vi "Clipper.vi"(8 "error in (no error)":errorcluster) -> (0 "error out":errorcluster)   [LabVIEW 2020]
doc: "This template is for the Queued Message Handler design pattern.\n\nThe Event Handling Loop generates messages based on user interface actions.\n\nThe Message Handling Loop processes messages generated by the Event Handling Loop, or by other messages. The messages are string values, so new messages can be added easily to the Message Cases case structure in the Message Handling Loop. Each message cluster can also provide an optional value for Message Data, which is a variant that can be converted to whatever message-specific data is required."
uses:
  <vilib>/Utility/miscctls.llb/LVCursorListTypeDef.ctl
  Analysis Support/Controls/UI Data-Clipper.ctl
  Collection Support/Message Queue/Enqueue Message (Single).vi
  Collection Support/Message Queue/Enqueue Message (Array).vi
  <vilib>/Utility/error.llb/Error Cluster From Error Code.vi
  <vilib>/ErrorRing/Error Ring.xnode
panel:
  in  "Stop Everything?":bool
  out "Right":dbl
  out "Left":dbl
  out "Flow":dynamicdata(graph)
  out "Pressure":dynamicdata(graph)
  out "Audio":dynamicdata(graph)
  out "File Name Display":string
  in  "Remove":bool
  in  "Set Cursors":bool
  in  "Edit File":bool
  out "Message":string
  in  "Save":bool
  in  "Open":bool
  in  "Exit":bool
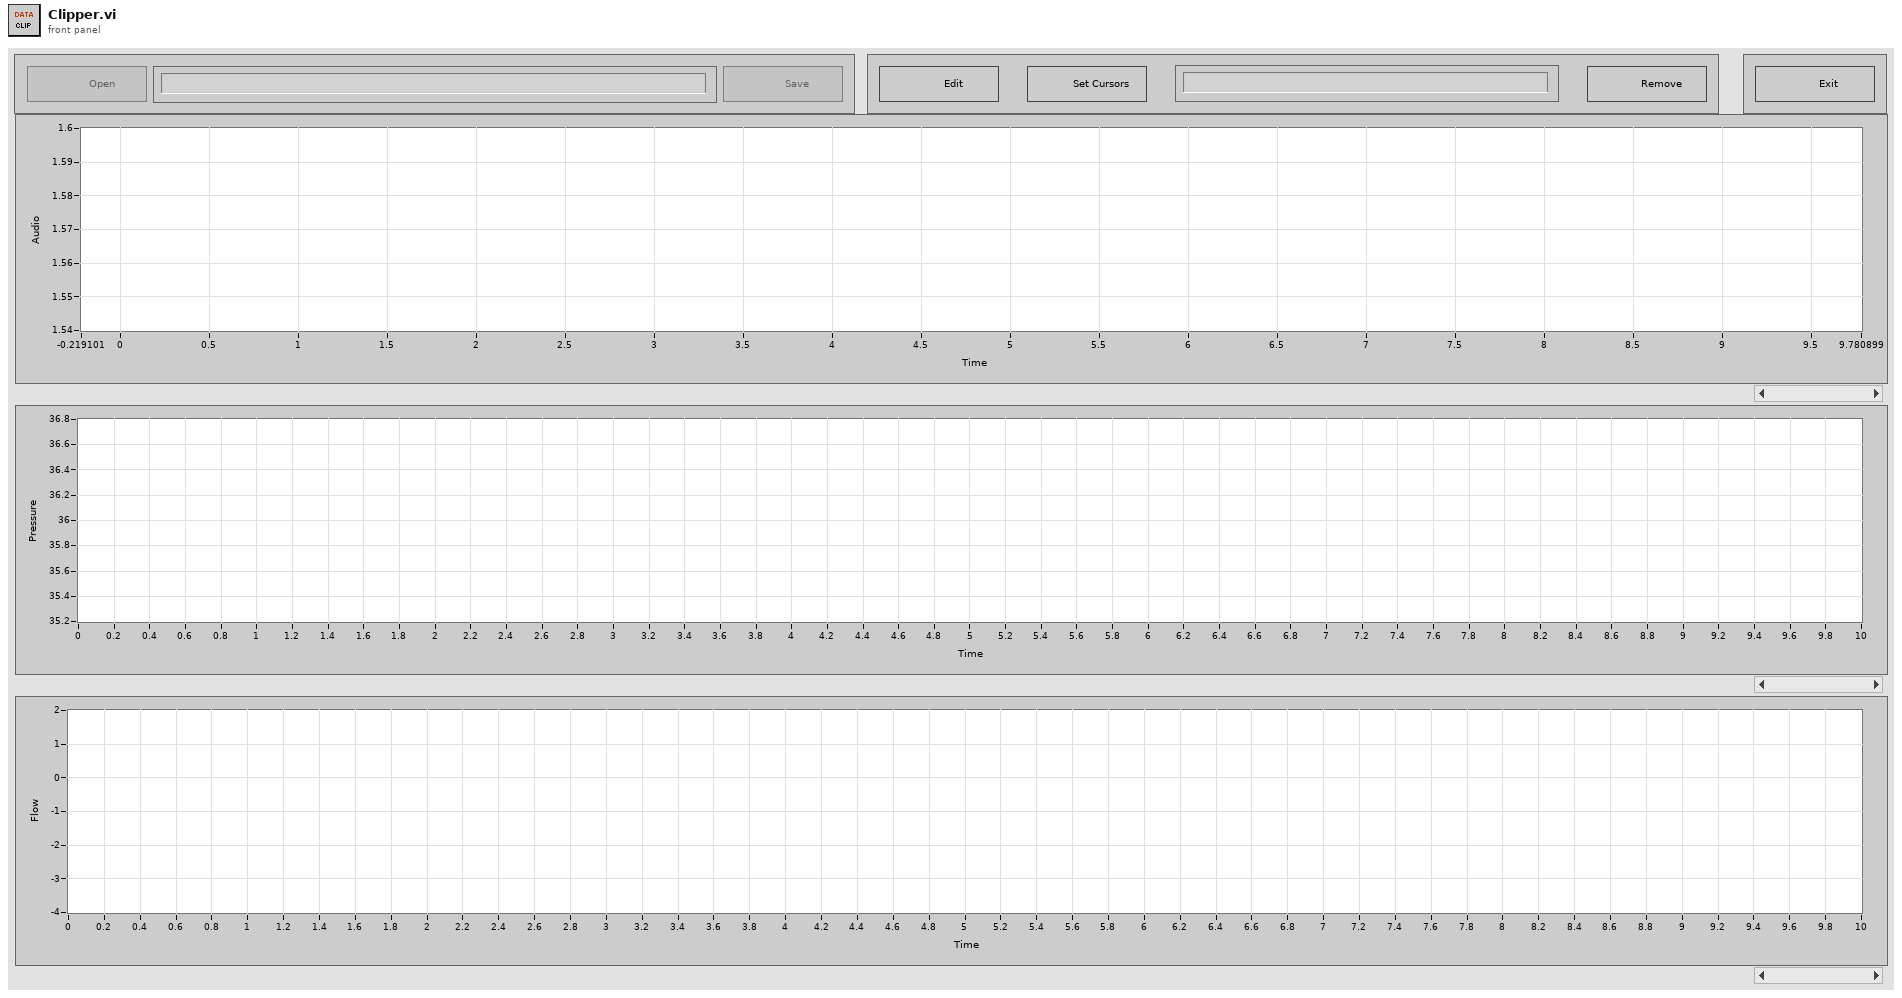
[diagram p1: front panel]
types:
  T1 = typedef "UI Data-Clipper.ctl" = cluster{"File Loaded?":bool, "Message":string, "Open Ref":refnum<vi>, "Save Ref":refnum<vi>, "Message Ref":refnum<vi>, "Exit Button Ref":refnum<vi>, "Remove Ref":refnum<vi>, "Set Cursors Ref":refnum<vi>, "Edit File Ref":refnum<vi>, "Audio Ref":refnum<vi>, "Pressure Ref":refnum<vi>, "Flow Ref":refnum<vi>, "Audio":dynamicdata, "Pressure":dynamicdata, "Flow":dynamicdata, "Left Cursor Position":dbl, "Right Cursor Position":dbl, "Cursors Locked?":bool, "File Name Display":string}
  T2 = typedef "LVCursorListTypeDef.ctl" = cluster{"Name":string, "Color":u32, "Style":u8, "Point Style":u8, "Name Visible":bool, "Allow Drag":bool, "Cursor Mode":u32, "Plot":i32, "Index":i32, "Position":cluster{"X":dbl, "Y":dbl}, "X Scale":u32, "Y Scale":u32, "Watch Plots":i32[], "Watch All Plots":bool, "Plot Area":i32, "Label Offset":cluster{"X":dbl, "Y":dbl}}[]
  T3 = typedef "All Message Queues.ctl" = cluster{"UI":refnum<queue>}
  T4 = cluster{"Cursor Constants[0]":cluster{"Name":string, "Color":u32, "Style":u8, "Point Style":u8, "Name Visible":bool, "Allow Drag":bool, "Cursor Mode":u32, "Plot":i32, "Index":i32, "Position":cluster{"X":dbl, "Y":dbl}, "X Scale":u32, "Y Scale":u32, "Watch Plots":i32[], "Watch All Plots":bool, "Plot Area":i32, "Label Offset":cluster{"X":dbl, "Y":dbl}}, "Cursor Constants[1]":cluster{"Name":string, "Color":u32, "Style":u8, "Point Style":u8, "Name Visible":bool, "Allow Drag":bool, "Cursor Mode":u32, "Plot":i32, "Index":i32, "Position":cluster{"X":dbl, "Y":dbl}, "X Scale":u32, "Y Scale":u32, "Watch Plots":i32[], "Watch All Plots":bool, "Plot Area":i32, "Label Offset":cluster{"X":dbl, "Y":dbl}}, "Cursor Constants[2]":cluster{"Name":string, "Color":u32, "Style":u8, "Point Style":u8, "Name Visible":bool, "Allow Drag":bool, "Cursor Mode":u32, "Plot":i32, "Index":i32, "Position":cluster{"X":dbl, "Y":dbl}, "X Scale":u32, "Y Scale":u32, "Watch Plots":i32[], "Watch All Plots":bool, "Plot Area":i32, "Label Offset":cluster{"X":dbl, "Y":dbl}}, "Cursor Constants[3]":cluster{"Name":string, "Color":u32, "Style":u8, "Point Style":u8, "Name Visible":bool, "Allow Drag":bool, "Cursor Mode":u32, "Plot":i32, "Index":i32, "Position":cluster{"X":dbl, "Y":dbl}, "X Scale":u32, "Y Scale":u32, "Watch Plots":i32[], "Watch All Plots":bool, "Plot Area":i32, "Label Offset":cluster{"X":dbl, "Y":dbl}}, "Cursor Constants[4]":cluster{"Name":string, "Color":u32, "Style":u8, "Point Style":u8, "Name Visible":bool, "Allow Drag":bool, "Cursor Mode":u32, "Plot":i32, "Index":i32, "Position":cluster{"X":dbl, "Y":dbl}, "X Scale":u32, "Y Scale":u32, "Watch Plots":i32[], "Watch All Plots":bool, "Plot Area":i32, "Label Offset":cluster{"X":dbl, "Y":dbl}}, "Cursor Constants[5]":cluster{"Name":string, "Color":u32, "Style":u8, "Point Style":u8, "Name Visible":bool, "Allow Drag":bool, "Cursor Mode":u32, "Plot":i32, "Index":i32, "Position":cluster{"X":dbl, "Y":dbl}, "X Scale":u32, "Y Scale":u32, "Watch Plots":i32[], "Watch All Plots":bool, "Plot Area":i32, "Label Offset":cluster{"X":dbl, "Y":dbl}}, "Cursor Constants[6]":cluster{"Name":string, "Color":u32, "Style":u8, "Point Style":u8, "Name Visible":bool, "Allow Drag":bool, "Cursor Mode":u32, "Plot":i32, "Index":i32, "Position":cluster{"X":dbl, "Y":dbl}, "X Scale":u32, "Y Scale":u32, "Watch Plots":i32[], "Watch All Plots":bool, "Plot Area":i32, "Label Offset":cluster{"X":dbl, "Y":dbl}}, "Cursor Constants[7]":cluster{"Name":string, "Color":u32, "Style":u8, "Point Style":u8, "Name Visible":bool, "Allow Drag":bool, "Cursor Mode":u32, "Plot":i32, "Index":i32, "Position":cluster{"X":dbl, "Y":dbl}, "X Scale":u32, "Y Scale":u32, "Watch Plots":i32[], "Watch All Plots":bool, "Plot Area":i32, "Label Offset":cluster{"X":dbl, "Y":dbl}}, "Cursor Constants[8]":cluster{"Name":string, "Color":u32, "Style":u8, "Point Style":u8, "Name Visible":bool, "Allow Drag":bool, "Cursor Mode":u32, "Plot":i32, "Index":i32, "Position":cluster{"X":dbl, "Y":dbl}, "X Scale":u32, "Y Scale":u32, "Watch Plots":i32[], "Watch All Plots":bool, "Plot Area":i32, "Label Offset":cluster{"X":dbl, "Y":dbl}}}
  T5 = cluster{"Name":string, "Color":u32, "Style":u8, "Point Style":u8, "Name Visible":bool, "Allow Drag":bool, "Cursor Mode":u32, "Plot":i32, "Index":i32, "Position":cluster{"X":dbl, "Y":dbl}, "X Scale":u32, "Y Scale":u32, "Watch Plots":i32[], "Watch All Plots":bool, "Plot Area":i32, "Label Offset":cluster{"X":dbl, "Y":dbl}}[]
  T6 = cluster{"CrsrList[0]":cluster{"Name":string, "Color":u32, "Style":u8, "Point Style":u8, "Name Visible":bool, "Allow Drag":bool, "Cursor Mode":u32, "Plot":i32, "Index":i32, "Position":cluster{"X":dbl, "Y":dbl}, "X Scale":u32, "Y Scale":u32, "Watch Plots":i32[], "Watch All Plots":bool, "Plot Area":i32, "Label Offset":cluster{"X":dbl, "Y":dbl}}, "CrsrList[1]":cluster{"Name":string, "Color":u32, "Style":u8, "Point Style":u8, "Name Visible":bool, "Allow Drag":bool, "Cursor Mode":u32, "Plot":i32, "Index":i32, "Position":cluster{"X":dbl, "Y":dbl}, "X Scale":u32, "Y Scale":u32, "Watch Plots":i32[], "Watch All Plots":bool, "Plot Area":i32, "Label Offset":cluster{"X":dbl, "Y":dbl}}, "CrsrList[2]":cluster{"Name":string, "Color":u32, "Style":u8, "Point Style":u8, "Name Visible":bool, "Allow Drag":bool, "Cursor Mode":u32, "Plot":i32, "Index":i32, "Position":cluster{"X":dbl, "Y":dbl}, "X Scale":u32, "Y Scale":u32, "Watch Plots":i32[], "Watch All Plots":bool, "Plot Area":i32, "Label Offset":cluster{"X":dbl, "Y":dbl}}, "CrsrList[3]":cluster{"Name":string, "Color":u32, "Style":u8, "Point Style":u8, "Name Visible":bool, "Allow Drag":bool, "Cursor Mode":u32, "Plot":i32, "Index":i32, "Position":cluster{"X":dbl, "Y":dbl}, "X Scale":u32, "Y Scale":u32, "Watch Plots":i32[], "Watch All Plots":bool, "Plot Area":i32, "Label Offset":cluster{"X":dbl, "Y":dbl}}, "CrsrList[4]":cluster{"Name":string, "Color":u32, "Style":u8, "Point Style":u8, "Name Visible":bool, "Allow Drag":bool, "Cursor Mode":u32, "Plot":i32, "Index":i32, "Position":cluster{"X":dbl, "Y":dbl}, "X Scale":u32, "Y Scale":u32, "Watch Plots":i32[], "Watch All Plots":bool, "Plot Area":i32, "Label Offset":cluster{"X":dbl, "Y":dbl}}, "CrsrList[5]":cluster{"Name":string, "Color":u32, "Style":u8, "Point Style":u8, "Name Visible":bool, "Allow Drag":bool, "Cursor Mode":u32, "Plot":i32, "Index":i32, "Position":cluster{"X":dbl, "Y":dbl}, "X Scale":u32, "Y Scale":u32, "Watch Plots":i32[], "Watch All Plots":bool, "Plot Area":i32, "Label Offset":cluster{"X":dbl, "Y":dbl}}, "CrsrList[6]":cluster{"Name":string, "Color":u32, "Style":u8, "Point Style":u8, "Name Visible":bool, "Allow Drag":bool, "Cursor Mode":u32, "Plot":i32, "Index":i32, "Position":cluster{"X":dbl, "Y":dbl}, "X Scale":u32, "Y Scale":u32, "Watch Plots":i32[], "Watch All Plots":bool, "Plot Area":i32, "Label Offset":cluster{"X":dbl, "Y":dbl}}, "CrsrList[7]":cluster{"Name":string, "Color":u32, "Style":u8, "Point Style":u8, "Name Visible":bool, "Allow Drag":bool, "Cursor Mode":u32, "Plot":i32, "Index":i32, "Position":cluster{"X":dbl, "Y":dbl}, "X Scale":u32, "Y Scale":u32, "Watch Plots":i32[], "Watch All Plots":bool, "Plot Area":i32, "Label Offset":cluster{"X":dbl, "Y":dbl}}, "CrsrList[8]":cluster{"Name":string, "Color":u32, "Style":u8, "Point Style":u8, "Name Visible":bool, "Allow Drag":bool, "Cursor Mode":u32, "Plot":i32, "Index":i32, "Position":cluster{"X":dbl, "Y":dbl}, "X Scale":u32, "Y Scale":u32, "Watch Plots":i32[], "Watch All Plots":bool, "Plot Area":i32, "Label Offset":cluster{"X":dbl, "Y":dbl}}}
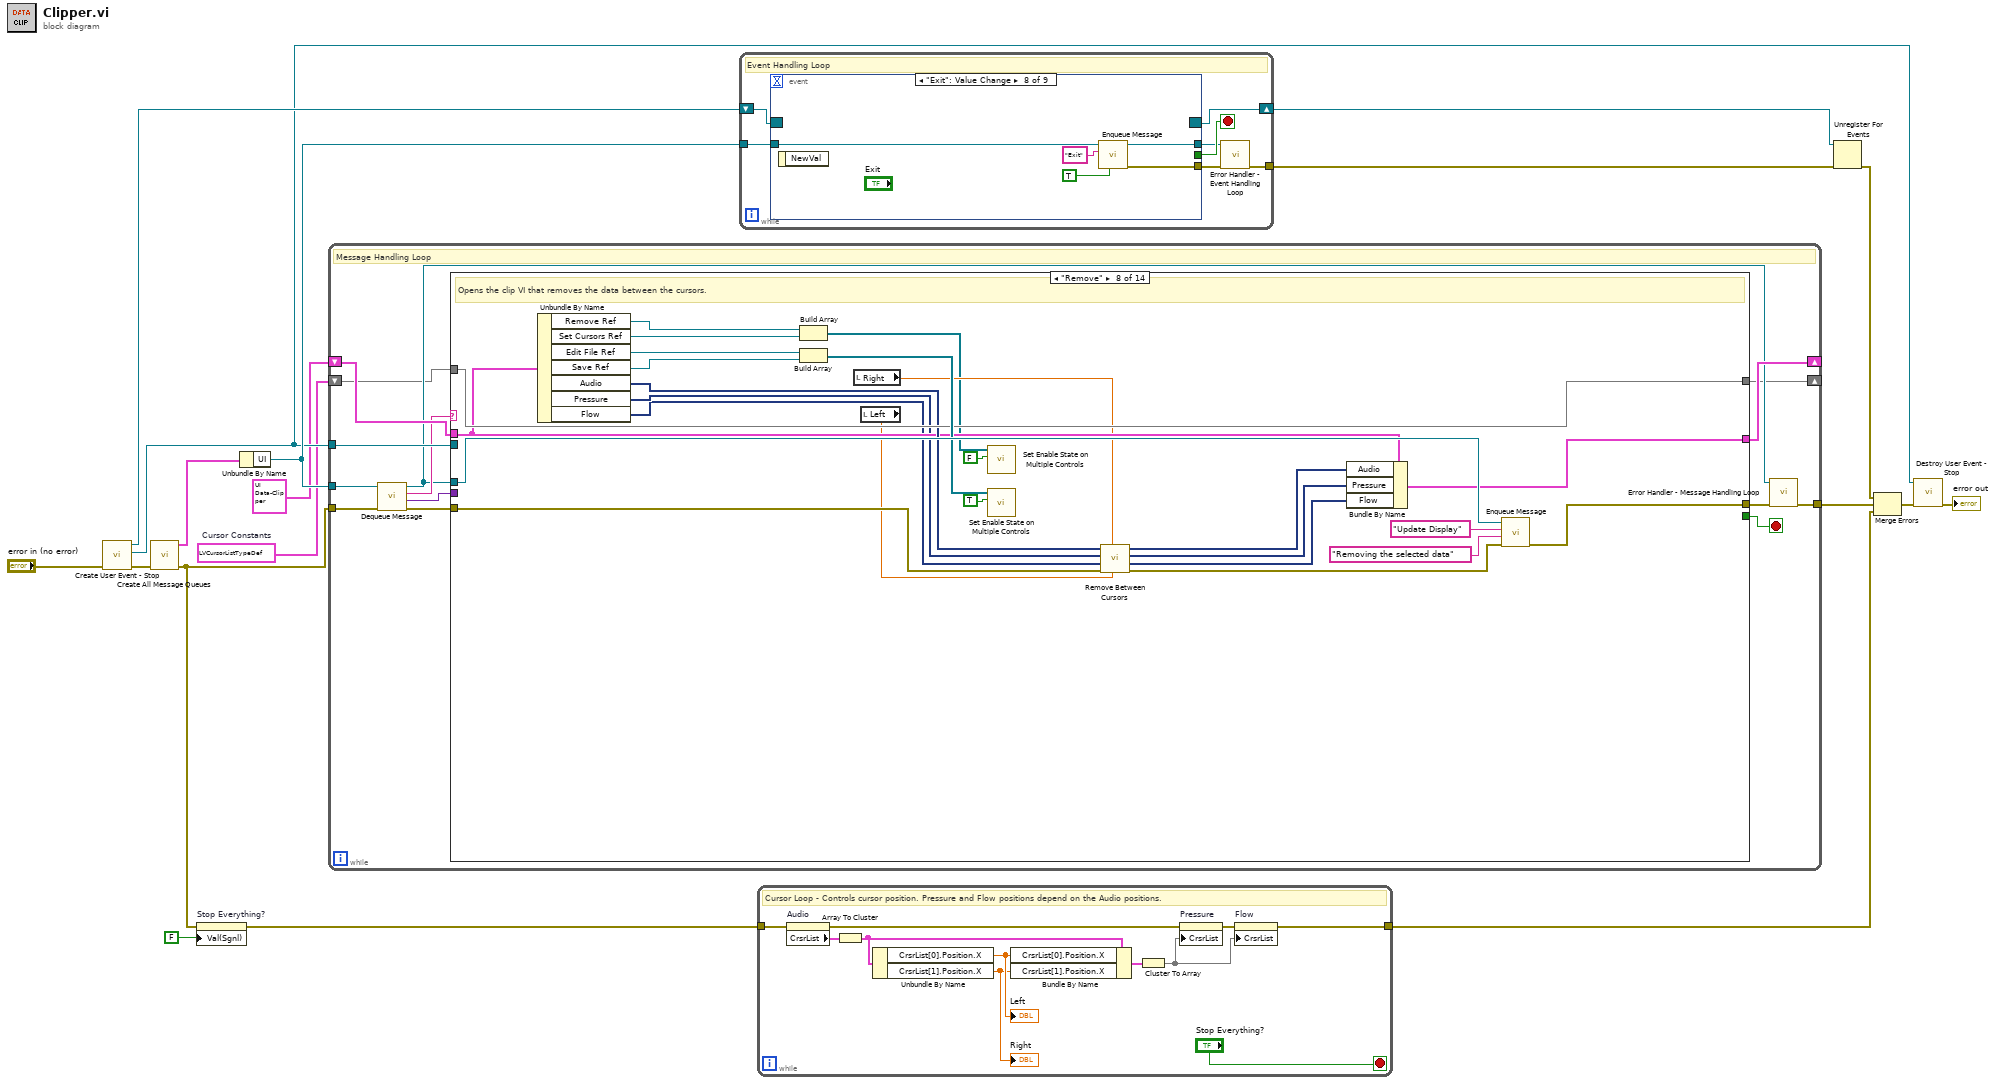
[diagram p0: block diagram]
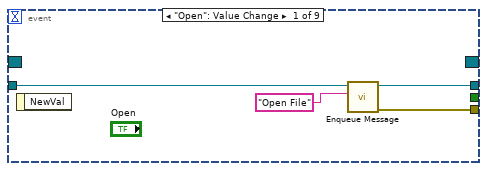
[diagram p2: hidden frame]
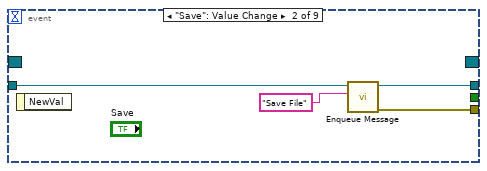
[diagram p3: hidden frame]
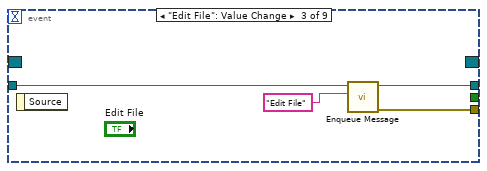
[diagram p4: hidden frame]
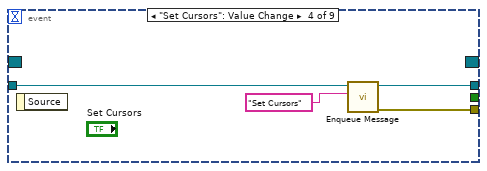
[diagram p5: hidden frame]
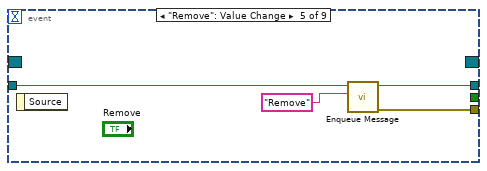
[diagram p6: hidden frame]
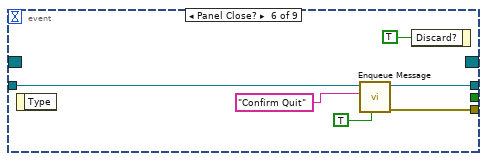
[diagram p7: hidden frame]
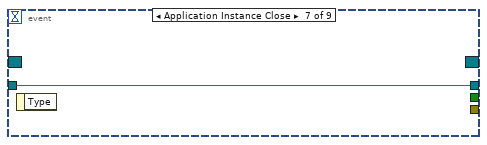
[diagram p8: hidden frame]
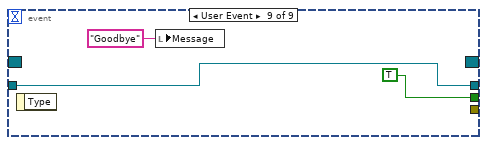
[diagram p9: hidden frame]
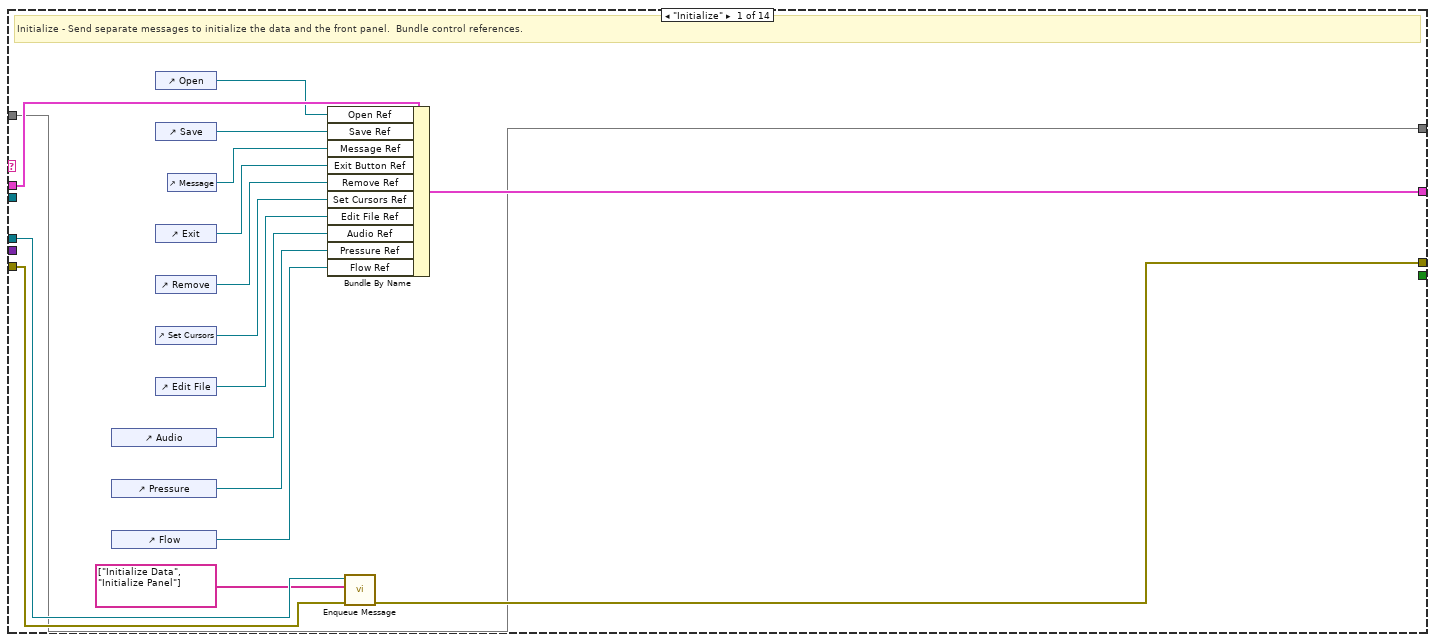
[diagram p10: hidden frame]
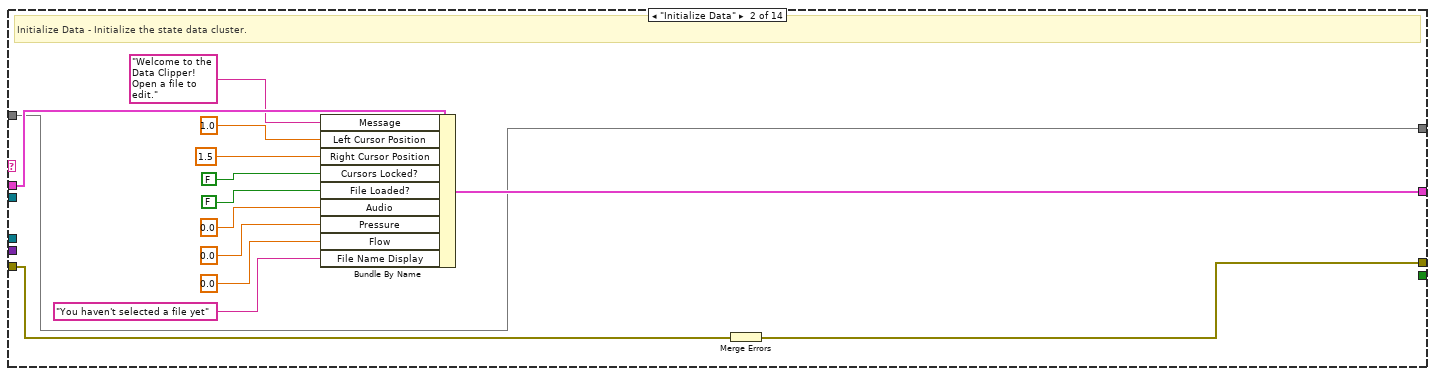
[diagram p11: hidden frame]
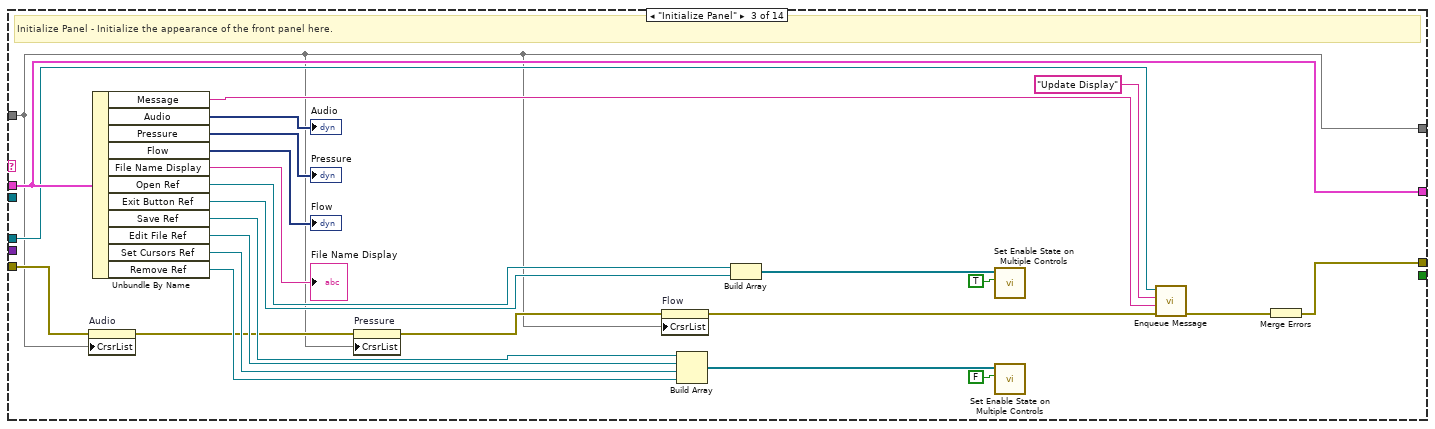
[diagram p12: hidden frame]
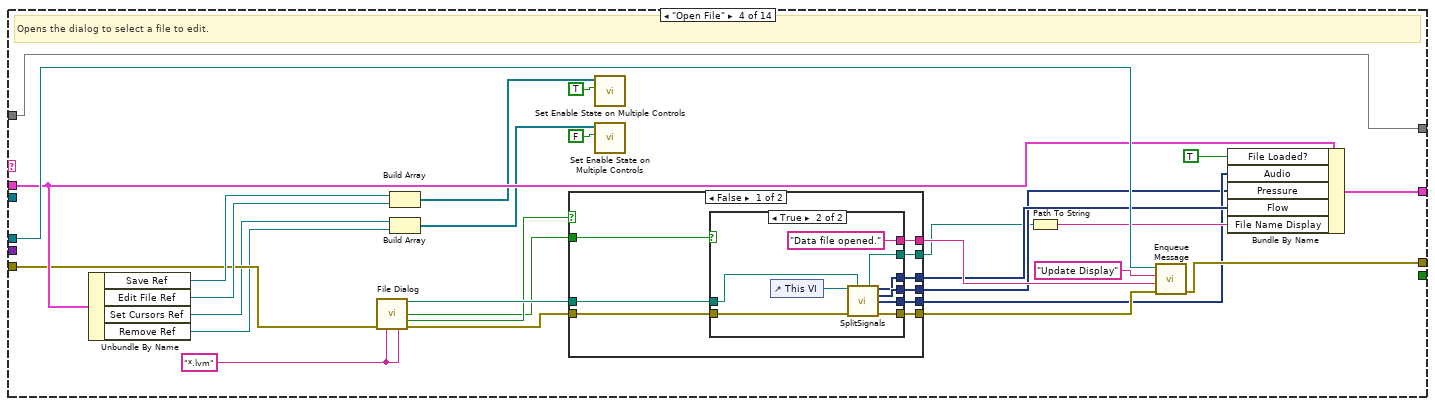
[diagram p13: hidden frame]
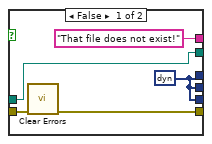
[diagram p14: hidden frame]
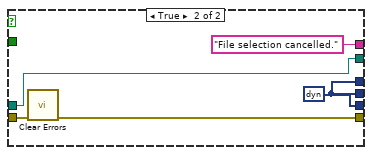
[diagram p15: hidden frame]
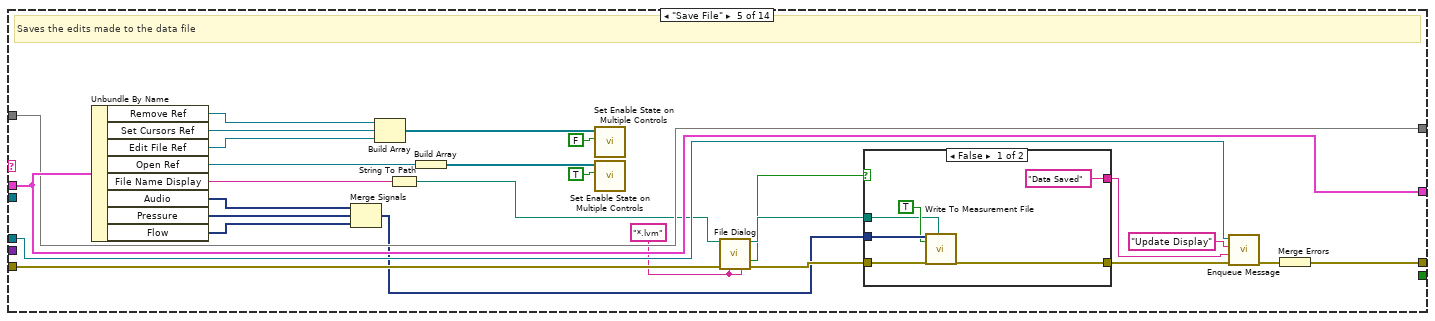
[diagram p16: hidden frame]
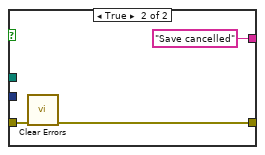
[diagram p17: hidden frame]
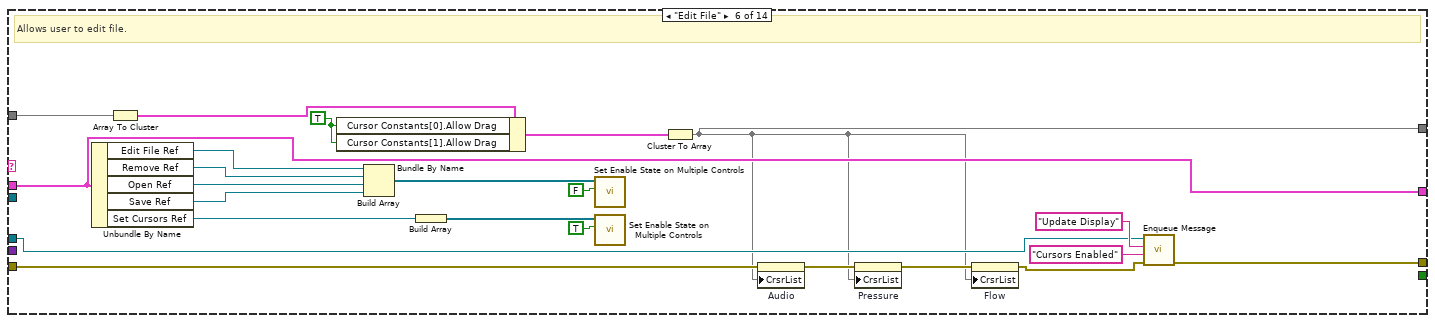
[diagram p18: hidden frame]
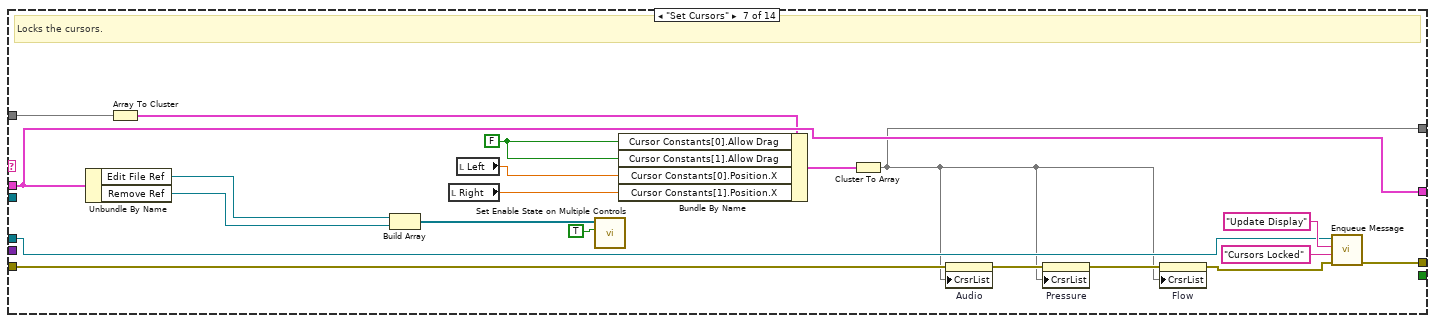
[diagram p19: hidden frame]
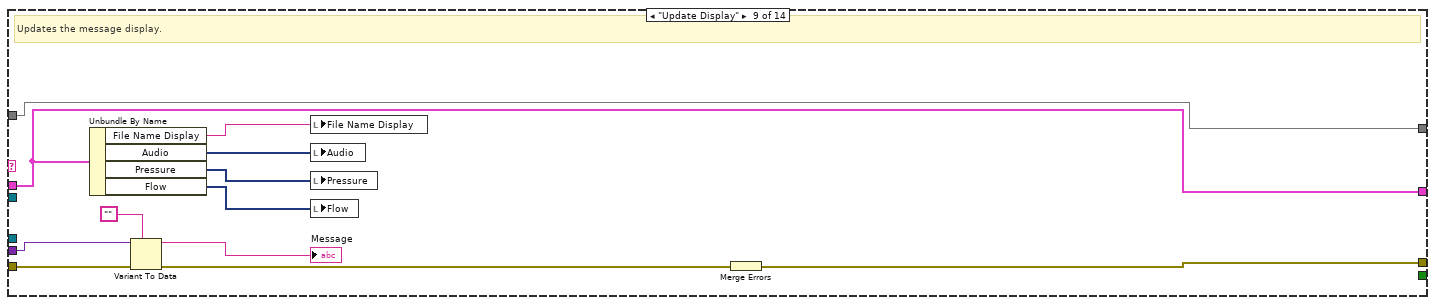
[diagram p20: hidden frame]
diagram:
  w9 = T2 [{"Name"="Left", "Color"=255, "Style"=2, "Point Style"=1, "Name Visible"=FALSE, "Allow Drag"=FALSE, "Cursor Mode"=0, "Plot"=0, "Index"=0, "Position"={"X"=2.0, "Y"=0.0}, "X Scale"=0, "Y Scale"=0, "Watch Plots"=[], "Watch All Plots"=FALSE, "Plot Area"=0, "Label Offset"={"X"=0.0, "Y"=0.0}}, {"Name"="Right", "Color"=13107455, "Style"=2, "Point Style"=1, "Name Visible"=FALSE, "Allow Drag"=FALSE, "Cursor Mode"=0, "Plot"=0, "Index"=0, "Position"={"X"=3.0, "Y"=0.0}, "X Scale"=0, "Y Scale"=0, "Watch Plots"=[], "Watch All Plots"=FALSE, "Plot Area"=0, "Label Offset"={"X"=0.0, "Y"=0.0}}]  # Cursor Constants
  n1 = call "Create User Event - Stop.vi"("error in (no error)"="error in (no error)") -> ("error out"=w8:errorcluster, "User Event - Stop"=w14:refnum<user-event>, "Stop Event Registration Refnum"=w15:refnum<event-registration>)  [unwired: 8 in]
  n2 = call "Create All Message Queues.vi"("error in (no error)"=w8) -> ("error out"=w5:errorcluster, "Message Queues out"=w18:T3)  [unwired: 9 in]
  n3 = property on="Stop Everything?" class="Bool (strict)"(error in=w5, "Val(Sgnl)"=FALSE ("Value (Signaling)")) -> (error out=w6:errorcluster)  [unwired: 1 in, 1 out]
  n4 = Unbundle By Name(w18) -> ("UI"=w16:refnum<queue>)
  n5 = while {
    tunnel: w16 -> [w24]
    shift-right: [w31] -> _
    shift-left: T1 {"File Loaded?"=FALSE, "Message"="", "Open Ref"=refnum, "Save Ref"=refnum, "Message Ref"=refnum, "Exit Button Ref"=refnum, "Remove Ref"=refnum, "Set Cursors Ref"=refnum, "Edit File Ref"=refnum, "Audio Ref"=refnum, "Pressure Ref"=refnum, "Flow Ref"=refnum, "Audio"=[], "Pressure"=[], "Flow"=[], "Left Cursor Position"=0.0, "Right Cursor Position"=0.0, "Cursors Locked?"=FALSE, "File Name Display"=""} ("UI Data") -> [w32]
    tunnel: w14 -> [w29]
    tunnel: w5 -> [w28]
    tunnel: [w22] -> w17
    shift-right: [w19] -> _
    shift-left: w9 -> [w20]
    stop <- w30 stop-if-true
    # "Message Handling Loop"
    n6 = call "Dequeue Message.vi"("error in (no error)"=w28, "Message Queue"=w24) -> ("error out"=w27:errorcluster, "Message Data"=w25:variant, "Message"=w26:string, "dup Message Queue"=w23:refnum<queue>)  [unwired: 6 in]
    n7 = case "Message Cases" shown="\"Remove\"" w26 {
      selector: w26 -> [_ _ _ _ _ _ _ _ _ _ _ _ _ w296]
      tunnel: w23 -> [w47 _ w86 w116 w169 w201 w221 w245 _ w264 w276 _ w294 _]
      tunnel: w27 -> [w48 w63 w66 w102 w156 w183 w207 w234 w259 w272 w280 w284 w289 _]
      tunnel: [w49 w51 w87 w93 w171 w200 w220 w246 w260 w265 w278 w282 w290 w297] -> w21
      tunnel: w32 -> [w46 w62 w88 w113 w167 w191 w217 w238 w254 w271 w279 w283 w293 w298]
      tunnel: [w45 w61 w88 w111 w167 w191 w217 w237 w254 w271 w279 w283 w293 w298] -> w31
      tunnel: [_ _ _ _ _ _ _ _ _ _ _ _ TRUE _] -> w30
      tunnel: w25 -> [_ _ _ _ _ _ _ _ w258 w270 _ _ _ _]
      tunnel: w29 -> [_ _ _ _ _ _ _ _ _ _ _ _ w288 _]
      tunnel: w20 -> [w33 w50 w64 w98 w158 w189 w211 w240 w249 w261 w273 w281 w285 w295]
      tunnel: [w33 w50 w64 w98 w158 w182 w206 w240 w249 w261 w273 w281 w285 w295] -> w19
      frame "Initialize" {
        # "Initialize - Send separate messages to initialize the data and the front panel.  Bundle control references."
        n8 = control-ref of="Audio"() -> (w37:refnum<vi>)
        n9 = control-ref of="Pressure"() -> (w36:refnum<vi>)
        n10 = control-ref of="Flow"() -> (w34:refnum<vi>)
        n11 = control-ref of="Open"() -> (w35:refnum<vi>)
        n12 = control-ref of="Save"() -> (w43:refnum<vi>)
        n13 = control-ref of="Exit"() -> (w41:refnum<vi>)
        n14 = control-ref of="Remove"() -> (w40:refnum<vi>)
        n15 = control-ref of="Set Cursors"() -> (w39:refnum<vi>)
        n16 = control-ref of="Edit File"() -> (w38:refnum<vi>)
        n17 = control-ref of="Message"() -> (w42:refnum<vi>)
        n18 = Bundle By Name(cluster=w46, "Open Ref"=w35, "Save Ref"=w43, "Message Ref"=w42, "Exit Button Ref"=w41, "Remove Ref"=w40, "Set Cursors Ref"=w39, "Edit File Ref"=w38, "Audio Ref"=w37, "Pressure Ref"=w36, "Flow Ref"=w34) -> (w45:T1)
        n19 = call-poly "Enqueue Message.vi"("error in (no error)"=w48, "Message Array"=string[] ["Initialize Data", "Initialize Panel"], "Message Queue"=w47) -> ("error out"=w49:errorcluster)  [unwired: 7 in, 1 out]
      }
      frame "Initialize Data" {
        # "Initialize Data - Initialize the state data cluster."
        n20 = Bundle By Name(cluster=w62, "Message"="Welcome to the Data Clipper! Open a file to edit." ("Initial Message"), "Left Cursor Position"=1.0, "Right Cursor Position"=1.5, "Cursors Locked?"=FALSE, "File Loaded?"=FALSE, "Audio"=0.0, "Pressure"=0.0, "Flow"=0.0, "File Name Display"="You haven't selected a file yet") -> (w61:T1)
        n21 = Merge Errors(w63) -> (w51:errorcluster)
      }
      frame "Initialize Panel" {
        # "Initialize Panel - Initialize the appearance of the front panel here."
        n22 = property on="Audio" class="WFGraph (strict)"(error in=w66, "CrsrList"=w64) -> (error out=w68:errorcluster)  [unwired: 1 in, 1 out]
        n23 = Unbundle By Name(w88) -> ("Message"=w70:string, "Audio"=→"Audio":dynamicdata, "Pressure"=→"Pressure":dynamicdata, "Flow"=→"Flow":dynamicdata, "File Name Display"=→"File Name Display":string, "Open Ref"=w78:refnum<vi>, "Exit Button Ref"=w77:refnum<vi>, "Save Ref"=w76:refnum<vi>, "Edit File Ref"=w75:refnum<vi>, "Set Cursors Ref"=w74:refnum<vi>, "Remove Ref"=w73:refnum<vi>)
        n24 = property on="Pressure" class="WFGraph (strict)"(error in=w68, "CrsrList"=w64) -> (error out=w67:errorcluster)  [unwired: 1 in, 1 out]
        n25 = property on="Flow" class="WFGraph (strict)"(error in=w67, "CrsrList"=w64) -> (error out=w65:errorcluster)  [unwired: 1 in, 1 out]
        n26 = Build Array(w76, w75, w74, w73) -> (w72:refnum<vi>[])
        n27 = Build Array(w78, w77) -> (w79:refnum<vi>[])
        n28 = call "Set Enable State on Multiple Controls.vi"("Enable?"=TRUE, "Controls"=w79) -> ()  [unwired: 10 in]
        n29 = call "Set Enable State on Multiple Controls.vi"("Enable?"=FALSE, "Controls"=w72) -> ()  [unwired: 10 in]
        n30 = call-poly "Enqueue Message.vi"("error in (no error)"=w65, "Message Data"=w70, "Message"="Update Display", "Message Queue"=w86) -> ("error out"=w85:errorcluster)  [unwired: 6 in, 1 out]
        n31 = Merge Errors(w85) -> (w87:errorcluster)
      }
      frame "Open File" {
        w106 = "*.lvm" ("pattern label")
        # "Opens the dialog to select a file to edit."
        n32 = Unbundle By Name(w113) -> ("Save Ref"=w108:refnum<vi>, "Edit File Ref"=w109:refnum<vi>, "Set Cursors Ref"=w97:refnum<vi>, "Remove Ref"=w94:refnum<vi>)
        n33 = call "File Dialog"("error in"=w102, "pattern (all files)"=w106, "pattern label"=w106) -> ("selected path"=w104:path, "exists"=w99:bool, "cancelled"=w100:bool, "error out"=w105:errorcluster)  [unwired: 9 in]
        n34 = Build Array(w108, w109) -> (w107:refnum<vi>[])
        n35 = Build Array(w97, w94) -> (w96:refnum<vi>[])
        n36 = case shown="False" w100 {
          tunnel: [w125 "File selection cancelled." ("\"Do Something\" button pressed")] -> w114
          tunnel: w105 -> [w124 w143]
          tunnel: w104 -> [w123 w140]
          tunnel: [w122 w142] -> w101
          tunnel: w99 -> [w121 _]
          tunnel: [w120 w141] -> w90
          tunnel: [w119 w141] -> w91
          tunnel: [w118 w141] -> w92
          tunnel: [w117 w140] -> w89
          frame False {
            n37 = case shown="True" w121 {
              tunnel: ["That file does not exist!" ("\"Do Something\" button pressed") "Data file opened." ("\"Do Something\" button pressed")] -> w125
              tunnel: w124 -> [w129 w138]
              tunnel: w123 -> [w126 w135]
              tunnel: [w128 w137] -> w122
              tunnel: [w127 w134] -> w120
              tunnel: [w127 w133] -> w119
              tunnel: [w127 w132] -> w118
              tunnel: [w126 w131] -> w117
              frame False {
                w127 = dynamicdata [] ("Waveform Graph")
                n38 = call <vilib>:"Clear Errors.vi"("error in (no error)"=w129) -> ("error out"=w128:errorcluster)  [unwired: 5 in, 1 out]
              }
              frame True {
                n39 = control-ref of="This VI"() -> (w136:refnum<vi>)
                n40 = call "SplitSignals.vi"("VI reference"=w136, "Filename"=w135, "Error In"=w138) -> ("Filename Out"=w131:path, "Flow"=w132:dynamicdata, "Pressure"=w134:dynamicdata, "Audio"=w133:dynamicdata, "Error Out"=w137:errorcluster)  [unwired: 5 in, 3 out]
              }
            }
          }
          frame True {
            w141 = dynamicdata [] ("Waveform Graph")
            n41 = call <vilib>:"Clear Errors.vi"("error in (no error)"=w143) -> ("error out"=w142:errorcluster)  [unwired: 5 in, 1 out]
          }
        }
        n42 = call "Set Enable State on Multiple Controls.vi"("Enable?"=TRUE, "Controls"=w107) -> ()  [unwired: 10 in]
        n43 = call "Set Enable State on Multiple Controls.vi"("Enable?"=FALSE, "Controls"=w96) -> ()  [unwired: 10 in]
        n44 = Path To String(path=w89) -> (string=w103:string)
        n45 = call-poly "Enqueue Message.vi"("error in (no error)"=w101, "Message Data"=w114, "Message"="Update Display", "Message Queue"=w116) -> ("error out"=w93:errorcluster)  [unwired: 6 in, 1 out]
        n46 = Bundle By Name(cluster=w113, "File Loaded?"=TRUE, "Audio"=w91, "Pressure"=w90, "Flow"=w92, "File Name Display"=w103) -> (w111:T1)
      }
      frame "Save File" {
        w154 = "*.lvm" ("pattern (all files)")
        # "Saves the edits made to the data file"
        n47 = Unbundle By Name(w167) -> ("Remove Ref"=w164:refnum<vi>, "Set Cursors Ref"=w163:refnum<vi>, "Edit File Ref"=w162:refnum<vi>, "Open Ref"=w159:refnum<vi>, "File Name Display"=w157:string, "Audio"=w151:dynamicdata, "Pressure"=w150:dynamicdata, "Flow"=w149:dynamicdata)
        n48 = Merge Signals(w151, w150, w149) -> (w148:dynamicdata)
        n49 = Build Array(w164, w163, w162) -> (w166:refnum<vi>[])
        n50 = String To Path(string=w157) -> (path=w155:path)
        n51 = Build Array(w159) -> (w161:refnum<vi>[])
        n52 = call "Set Enable State on Multiple Controls.vi"("Enable?"=FALSE, "Controls"=w166) -> ()  [unwired: 10 in]
        n53 = call "Set Enable State on Multiple Controls.vi"("Enable?"=TRUE, "Controls"=w161) -> ()  [unwired: 10 in]
        n54 = call "File Dialog"("start path"=w155, "error in"=w156, "pattern (all files)"=w154, "pattern label"=w154) -> ("selected path"=w147:path, "cancelled"=w146:bool, "error out"=w153:errorcluster)  [unwired: 8 in, 1 out]
        n55 = case shown="False" w146 {
          tunnel: w153 -> [w177 w179]
          tunnel: [w176 w178] -> w152
          tunnel: w148 -> [w175 _]
          tunnel: w147 -> [w173 _]
          tunnel: ["Data Saved" ("\"Do Something Else\" button pressed") "Save cancelled" ("\"Do Something Else\" button pressed")] -> w145
          frame False {
            n56 = call "Write To Measurement File"("Signals"=w175, "Reset"=TRUE, "error in (no error)"=w177, "Filename"=w173) -> ("error out"=w176:errorcluster)  [unwired: 13 in, 2 out]
          }
          frame True {
            n57 = call <vilib>:"Clear Errors.vi"("error in (no error)"=w179) -> ("error out"=w178:errorcluster)  [unwired: 5 in, 1 out]
          }
        }
        n58 = call-poly "Enqueue Message.vi"("error in (no error)"=w152, "Message Data"=w145, "Message"="Update Display", "Message Queue"=w169) -> ("error out"=w170:errorcluster)  [unwired: 6 in, 1 out]
        n59 = Merge Errors(w170) -> (w171:errorcluster)
      }
      frame "Edit File" {
        w190 = TRUE ("CrsrList[0].Allow Drag")
        # "Allows user to edit file."
        n60 = Unbundle By Name(w191) -> ("Edit File Ref"=w181:refnum<vi>, "Remove Ref"=w192:refnum<vi>, "Open Ref"=w197:refnum<vi>, "Save Ref"=w196:refnum<vi>, "Set Cursors Ref"=w193:refnum<vi>)
        n61 = Array To Cluster(array=w189) -> (cluster=w188:T4)
        n62 = Bundle By Name(cluster=w188, "Cursor Constants[0].Allow Drag"=w190, "Cursor Constants[1].Allow Drag"=w190) -> (w187:T4)
        n63 = Build Array(w181, w192, w197, w196) -> (w199:refnum<vi>[])
        n64 = Build Array(w193) -> (w195:refnum<vi>[])
        n65 = call "Set Enable State on Multiple Controls.vi"("Enable?"=FALSE, "Controls"=w199) -> ()  [unwired: 10 in]
        n66 = call "Set Enable State on Multiple Controls.vi"("Enable?"=TRUE, "Controls"=w195) -> ()  [unwired: 10 in]
        n67 = Cluster To Array(cluster=w187) -> (array=w182:T5)
        n68 = property on="Audio" class="WFGraph (strict)"(error in=w183, "CrsrList"=w182) -> (error out=w186:errorcluster)  [unwired: 1 in, 1 out]
        n69 = property on="Pressure" class="WFGraph (strict)"(error in=w186, "CrsrList"=w182) -> (error out=w185:errorcluster)  [unwired: 1 in, 1 out]
        n70 = property on="Flow" class="WFGraph (strict)"(error in=w185, "CrsrList"=w182) -> (error out=w184:errorcluster)  [unwired: 1 in, 1 out]
        n71 = call-poly "Enqueue Message.vi"("error in (no error)"=w184, "Message Data"="Cursors Enabled" ("\"Do Something Else\" button pressed"), "Message"="Update Display", "Message Queue"=w201) -> ("error out"=w200:errorcluster)  [unwired: 6 in, 1 out]
      }
      frame "Set Cursors" {
        w214 = FALSE ("CrsrList[0].Allow Drag")
        # "Locks the cursors."
        n72 = Unbundle By Name(w217) -> ("Edit File Ref"=w216:refnum<vi>, "Remove Ref"=w215:refnum<vi>)
        n73 = Array To Cluster(array=w211) -> (cluster=w212:T4)
        n74 = Build Array(w216, w215) -> (w219:refnum<vi>[])
        n75 = local read "Right"() -> (w204:dbl)
        n76 = local read "Left"() -> (w205:dbl)
        n77 = call "Set Enable State on Multiple Controls.vi"("Enable?"=TRUE, "Controls"=w219) -> ()  [unwired: 10 in]
        n78 = Bundle By Name(cluster=w212, "Cursor Constants[0].Allow Drag"=w214, "Cursor Constants[1].Allow Drag"=w214, "Cursor Constants[0].Position.X"=w205, "Cursor Constants[1].Position.X"=w204) -> (w213:T4)
        n79 = Cluster To Array(cluster=w213) -> (array=w206:T5)
        n80 = property on="Audio" class="WFGraph (strict)"(error in=w207, "CrsrList"=w206) -> (error out=w210:errorcluster)  [unwired: 1 in, 1 out]
        n81 = property on="Pressure" class="WFGraph (strict)"(error in=w210, "CrsrList"=w206) -> (error out=w209:errorcluster)  [unwired: 1 in, 1 out]
        n82 = property on="Flow" class="WFGraph (strict)"(error in=w209, "CrsrList"=w206) -> (error out=w208:errorcluster)  [unwired: 1 in, 1 out]
        n83 = call-poly "Enqueue Message.vi"("error in (no error)"=w208, "Message Data"="Cursors Locked" ("\"Do Something Else\" button pressed"), "Message"="Update Display", "Message Queue"=w221) -> ("error out"=w220:errorcluster)  [unwired: 6 in, 1 out]
      }
      frame "Remove" {
        # "Opens the clip VI that removes the data between the cursors."
        n84 = Unbundle By Name(w238) -> ("Remove Ref"=w224:refnum<vi>, "Set Cursors Ref"=w225:refnum<vi>, "Edit File Ref"=w242:refnum<vi>, "Save Ref"=w241:refnum<vi>, "Audio"=w239:dynamicdata, "Pressure"=w231:dynamicdata, "Flow"=w230:dynamicdata)
        n85 = Build Array(w224, w225) -> (w227:refnum<vi>[])
        n86 = Build Array(w242, w241) -> (w244:refnum<vi>[])
        n87 = local read "Right"() -> (w232:dbl)
        n88 = local read "Left"() -> (w233:dbl)
        n89 = call "Set Enable State on Multiple Controls.vi"("Enable?"=FALSE, "Controls"=w227) -> ()  [unwired: 10 in]
        n90 = call "Set Enable State on Multiple Controls.vi"("Enable?"=TRUE, "Controls"=w244) -> ()  [unwired: 10 in]
        n91 = call "Remove Between Cursors.vi"("Left"=w233, "Right"=w232, "error in (no error)"=w234, "Flow"=w230, "Pressure"=w231, "Audio"=w239) -> ("error out"=w235:errorcluster, "Flow Clipped"=w228:dynamicdata, "Pressure Clipped"=w229:dynamicdata, "Audio Clipped"=w236:dynamicdata)  [unwired: 2 in]
        n92 = Bundle By Name(cluster=w238, "Audio"=w236, "Pressure"=w229, "Flow"=w228) -> (w237:T1)
        n93 = call-poly "Enqueue Message.vi"("error in (no error)"=w235, "Message Data"="Removing the selected data" ("\"Do Something Else\" button pressed"), "Message"="Update Display", "Message Queue"=w245) -> ("error out"=w246:errorcluster)  [unwired: 6 in, 1 out]
      }
      frame "Update Display" {
        # "Updates the message display."
        n94 = Unbundle By Name(w254) -> ("File Name Display"=w253:string, "Audio"=w252:dynamicdata, "Pressure"=w251:dynamicdata, "Flow"=w250:dynamicdata)
        n95 = Variant To Data(error in=w259, type="", Variant=w258) -> (data=→"Message":string, error out=w256:errorcluster)
        n96 = local write "File Name Display"(w253) -> ()
        n97 = local write "Audio"(w252) -> ()
        n98 = local write "Pressure"(w251) -> ()
        n99 = local write "Flow"(w250) -> ()
        n100 = Merge Errors(w256) -> (w260:errorcluster)
      }
      frame "Error" {
        # "Error - Check the error message data and respond accordingly. This message is sent by the \"Error Handler\" VIs at the end of each loop in this application."
        n101 = Variant To Data(error in=w272, type=errorcluster {"status"=FALSE, "code"=0, "source"=""} ("error constant"), Variant=w270) -> (data=w268:errorcluster, error out=w267:errorcluster)
        n102 = call <vilib>:"Simple Error Handler.vi"("error in (no error)"=w268) -> ()  [unwired: 4 in, 5 out]
        n103 = call-poly "Enqueue Message.vi"("Priority Message? (F)"=TRUE, "Message"="Exit", "Message Queue"=w264) -> ("error out"=w266:errorcluster)  [unwired: 7 in, 1 out]
        n104 = Merge Errors(w266, w267) -> (w265:errorcluster)
      }
      frame "Confirm Quit" {
        # "Confirm Quit - Message that can confirm whether or not the user wants to exit the application."
        n105 = call-poly "Enqueue Message.vi"("Priority Message? (F)"=TRUE, "error in (no error)"=w280, "Message"="Exit", "Message Queue"=w276) -> ("error out"=w277:errorcluster)  [unwired: 6 in, 1 out]
        n106 = Merge Errors(w277) -> (w278:errorcluster)
      }
      frame "---Copy This Frame---" {
        # "Duplicate this frame when creating new messages.  Change this comment in the duplicated frame to describe this message."
        n107 = Merge Errors(w284) -> (w282:errorcluster)
      }
      frame "Exit" {
        # "Exit - Exit the application."
        n108 = Release Queue(queue=w294, error in (no error)=w289) -> (error out=w291:errorcluster)  [unwired: 1 in, 2 out]
        n109 = call "Fire User Event - Stop.vi"("User Event - Stop"=w288) -> ("error out"=w287:errorcluster)  [unwired: 10 in]
        n110 = Merge Errors(w287, w291) -> (w290:errorcluster)
        n111 = local write "Stop Everything?"(TRUE ("Stop Everything?")) -> ()
      }
      frame Default {
        # "'Default' case only runs if there is a message that isn't defined in any of the other cases.  Output a programming error."
        n112 = xnode "Error Ring"("parameter 0"=w296) -> ("error out"=w297:errorcluster)
      }
    }
    n113 = call "Error Handler - Message Handling Loop.vi"("error in (no error)"=w21, "Message Queue"=w23) -> ("dup error in"=w22:errorcluster)  [unwired: 8 in, 1 out]
  }
  n114 = while {
    tunnel: w16 -> [w312]
    shift-right: [w310] -> w12
    shift-left: w15 -> [w311]
    tunnel: [w306] -> w11
    stop <- w308 stop-if-true
    # "Event Handling Loop"
    n115 = event shown="[7] \"Exit\": Value Change" {
      selector: w311 -> [_ _ _ _ _ _ _ _ _]
      dyn-events: [_ _ _ _ _ _ _ _ _] -> w310
      timeout: _ -> [_ _ _ _ _ _ _ _ _]
      tunnel: [_ _ _ _ _ _ _ _ TRUE ("Discard?")] -> w308
      tunnel: w312 -> [w316 w320 w323 w327 w331 w337 w339 w344 w347]
      tunnel: [w313 w317 w322 w326 w329 w336 _ w343 _] -> w309
      tunnel: [w315 w319 w321 w325 w330 w335 w339 w342 w347] -> w307
      event "Open": Value Change {
        n116 = event-data() -> ()  [unwired: 1 in, 1 out]
        n117 = call-poly "Enqueue Message.vi"("Message"="Open File", "Message Queue"=w316) -> ("error out"=w313:errorcluster, "dup Message Queue"=w315:refnum<queue>)  [unwired: 8 in]
      }
      event "Save": Value Change {
        n118 = event-data() -> ()  [unwired: 1 in, 1 out]
        n119 = call-poly "Enqueue Message.vi"("Message"="Save File", "Message Queue"=w320) -> ("error out"=w317:errorcluster, "dup Message Queue"=w319:refnum<queue>)  [unwired: 8 in]
      }
      event "Edit File": Value Change {
        n120 = event-data() -> ()  [unwired: 1 in, 1 out]
        n121 = call-poly "Enqueue Message.vi"("Message"="Edit File", "Message Queue"=w323) -> ("error out"=w322:errorcluster, "dup Message Queue"=w321:refnum<queue>)  [unwired: 8 in]
      }
      event "Set Cursors": Value Change {
        n122 = event-data() -> ()  [unwired: 1 in, 1 out]
        n123 = call-poly "Enqueue Message.vi"("Message"="Set Cursors", "Message Queue"=w327) -> ("error out"=w326:errorcluster, "dup Message Queue"=w325:refnum<queue>)  [unwired: 8 in]
      }
      event "Remove": Value Change {
        n124 = event-data() -> ()  [unwired: 1 in, 1 out]
        n125 = call-poly "Enqueue Message.vi"("Message"="Remove", "Message Queue"=w331) -> ("error out"=w329:errorcluster, "dup Message Queue"=w330:refnum<queue>)  [unwired: 8 in]
      }
      event Panel Close? {
        n126 = event-data() -> ()  [unwired: 1 in, 1 out]
        n127 = call-poly "Enqueue Message.vi"("Priority Message? (F)"=TRUE, "Message"="Confirm Quit", "Message Queue"=w337) -> ("error out"=w336:errorcluster, "dup Message Queue"=w335:refnum<queue>)  [unwired: 7 in]
        n128 = event-data("Discard?"=TRUE) -> ()  [unwired: 1 in, 1 out]
      }
      event Application Instance Close {
        n129 = event-data() -> ()  [unwired: 1 in, 1 out]
      }
      event "Exit": Value Change {
        n130 = event-data() -> ()  [unwired: 1 in, 1 out]
        n131 = call-poly "Enqueue Message.vi"("Priority Message? (F)"=TRUE, "Message"="Exit", "Message Queue"=w344) -> ("error out"=w343:errorcluster, "dup Message Queue"=w342:refnum<queue>)  [unwired: 7 in]
      }
      event User Event {
        # "The Message Handling Loop processed an \"Exit\" message, which fired this event to stop the Event Handling Loop."
        n132 = event-data() -> ()  [unwired: 1 in, 1 out]
        n133 = local write "Message"("Goodbye" ("VI Stopped")) -> ()
      }
    }
    n134 = call "Error Handler - Event Handling Loop.vi"("error in (no error)"=w309, "Message Queue"=w307) -> ("dup error in"=w306:errorcluster)  [unwired: 8 in, 1 out]
  }
  n135 = while {
    tunnel: w6 -> [w354]
    tunnel: [w352] -> w10
    stop <- "Stop Everything?" stop-if-true
    # "Cursor Loop - Controls cursor position. Pressure and Flow positions depend on the Audio positions."
    n136 = property on="Audio" class="WFGraph (strict)"(error in=w354) -> (error out=w353:errorcluster, "CrsrList"=w355:T2)  [unwired: 1 in, 1 out]
    n137 = Array To Cluster(array=w355) -> (cluster=w350:T6)
    n138 = Unbundle By Name(w350) -> ("CrsrList[0].Position.X"=w357:dbl, "CrsrList[1].Position.X"=w351:dbl)
    "Left" <- w357
    "Right" <- w351
    n139 = Bundle By Name(cluster=w350, "CrsrList[0].Position.X"=w357, "CrsrList[1].Position.X"=w351) -> (w349:T6)
    n140 = Cluster To Array(cluster=w349) -> (array=w348:T5)
    n141 = property on="Pressure" class="WFGraph (strict)"(error in=w353, "CrsrList"=w348) -> (error out=w356:errorcluster)  [unwired: 1 in, 1 out]
    n142 = property on="Flow" class="WFGraph (strict)"(error in=w356, "CrsrList"=w348) -> (error out=w352:errorcluster)  [unwired: 1 in, 1 out]
  }
  n143 = Unregister For Events(event registration refnum=w12, error in=w11) -> (error out=w13:errorcluster)
  n144 = Merge Errors(w13, w17, w10) -> (w7:errorcluster)
  n145 = call "Destroy User Event - Stop.vi"("error in (no error)"=w7, "User Event - Stop"=w14) -> ("error out"=→"error out":errorcluster)  [unwired: 9 in]
